vi "SpectrumToColor.vi"(1 "Reflectance":dbl[](array[numeric]), 2 "CMF":dbl[][](array[numeric]), 3 "Illuminant":cluster{"String":string, "Array":dbl[]}, 4 "Selected RGB":string(combo)) -> (0 "Color,XYZ,RGB,Lab":T1)   [LabVIEW 2013]
panel:
  out "RGBStandardRows":i32
  out "RGBStandards":string[][](array[string])
  out "WhiteReference":i32[](array[numeric])
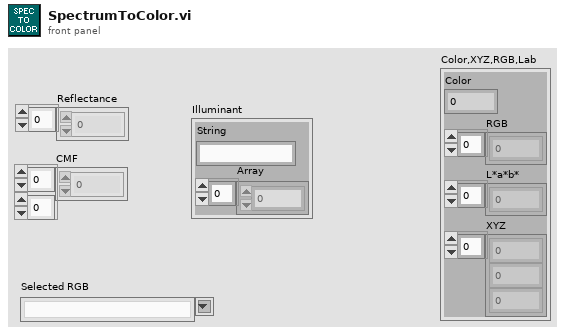
[diagram p1: front panel]
types:
  T1 = cluster{"Color":u32, "RGB":dbl[], "L*a*b*":dbl[], "XYZ":dbl[]}
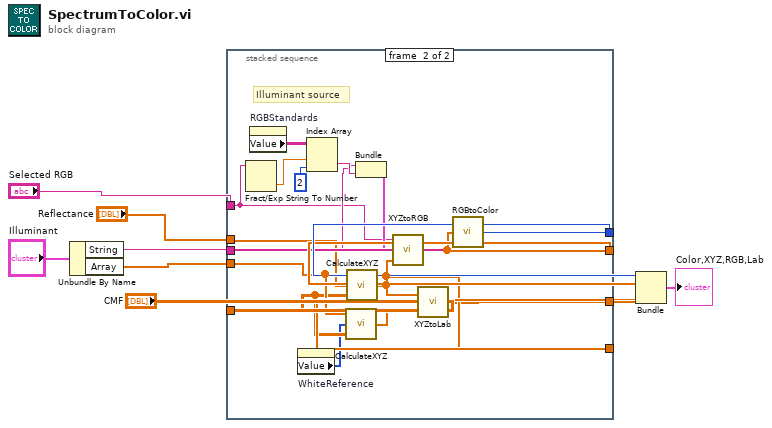
[diagram p0: block diagram]
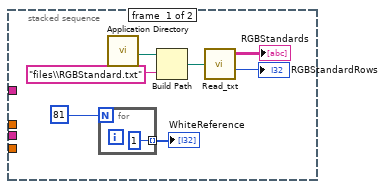
[diagram p2: hidden frame]
diagram:
  n1 = Unbundle By Name("Illuminant") -> ("String"=w1:string, "Array"=w2:dbl[])
  n2 = stacked-sequence {
    tunnel: w2 -> [_ w35]
    tunnel: "CMF" -> [_ w34]
    tunnel: [_ w24] -> w8
    tunnel: "Selected RGB" -> [_ w20]
    tunnel: [_ w22] -> w9
    tunnel: [_ w32] -> w10
    tunnel: [_ w31] -> w6
    tunnel: "Reflectance" -> [_ w30]
    tunnel: w1 -> [_ w25]
    frame #0 {
      n3 = for {
        N: 81 -> [_]
        tunnel: [1] -> w18 mode=indexing
      }
      "WhiteReference" <- w18
      n4 = call <vilib>:"Application Directory.vi"() -> ("Application Directory"=w12:path)
      n5 = Build Path(base path=w12, name or relative path="files\\RGBStandard.txt") -> (appended path=w13:path)
      n6 = call "Read_txt.vi"("file path (dialog if empty)"=w13) -> ("Elements"=→"RGBStandards":string[][], "Rows"=→"RGBStandardRows":i32)  [unwired: 1 out]
    }
    frame #1 {
      # "Illuminant source"
      n7 = Fract/Exp String To Number(string=w20) -> (number=w27:dbl)  [unwired: 3 in, 1 out]
      n8 = property on="RGBStandards" class="Arr (strict)"() -> ("Value"=w29:string[][])  [unwired: 2 in, 2 out]
      n9 = property on="WhiteReference" class="Arr (strict)"() -> ("Value"=w33:i32[])  [unwired: 2 in, 2 out]
      n10 = Index Array(array=w29, index (row)=w27, index (col)=2 ("disabled index (col)")) -> (element=w26:string)
      n11 = call "CalculateXYZ.vi"("CMF"=w34, "Reflectance"=w33, "Illuminant"=w35) -> ("XYZ"=w23:dbl[])
      n12 = call "CalculateXYZ.vi"("CMF"=w34, "Reflectance"=w30, "Illuminant"=w35) -> ("XYZ"=w31:dbl[])
      n13 = Bundle("String"=w25, "String"=w26) -> (w21:cluster{"String":string, "String":string})  [unwired: 1 in]
      n14 = call "XYZtoRGB.vi"("XYZ"=w31, "Illuminants"=w21, "Selected RGB"=w20) -> ("RGB"=w22:dbl[])
      n15 = call "XYZtoLab.vi"("XrYrZr"=w23, "XYZ"=w31) -> ("L*a*b*"=w24:dbl[])
      n16 = call "RGBtoColor.vi"("RGB"=w22) -> ("Color"=w32:u32)
    }
  }
  n17 = Bundle("Color"=w10, "RGB"=w9, "L*a*b*"=w8, "XYZ"=w6) -> (→"Color,XYZ,RGB,Lab":T1)  [unwired: 1 in]
